vi "Weather API test.vi"() -> ()   [LabVIEW 2019]
uses:
  Source/Open Weather Session/Public/Controls/Weather Data.ctl
  Source/Open Weather Session/Public/Controls/Weather Sample Data.ctl
  Source/Open Weather Session/Public/Controls/Weather Description Data.ctl
  Source/Open Weather Session/Public/Controls/Coordenates.ctl
  Source/Open Weather Session/Open Weather Session.lvclass
panel:
  out "Weather Data":T1
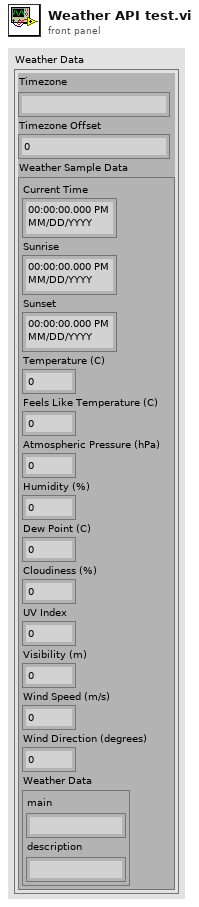
[diagram p1: front panel]
types:
  T1 = typedef "Open Weather Session.lvclass/Weather Data.ctl" = cluster{"Timezone":string, "Timezone Offset":dbl, "Weather Sample Data":T2}
  T2 = typedef "Open Weather Session.lvclass/Weather Sample Data.ctl" = cluster{"Current Time":timestamp, "Sunrise":timestamp, "Sunset":timestamp, "Temperature (C)":dbl, "Feels Like Temperature (C)":dbl, "Atmospheric Pressure (hPa)":dbl, "Humidity (%)":dbl, "Dew Point (C)":dbl, "Cloudiness (%)":dbl, "UV Index":dbl, "Visibility (m)":dbl, "Wind Speed (m/s)":dbl, "Wind Direction (degrees)":dbl, "Weather Data":T3}
  T3 = typedef "Open Weather Session.lvclass/Weather Description Data.ctl" = cluster{"main":string, "description":string}
  T4 = typedef "Open Weather Session.lvclass/Coordenates.ctl" = cluster{"Latitude":dbl, "Longitude":dbl}
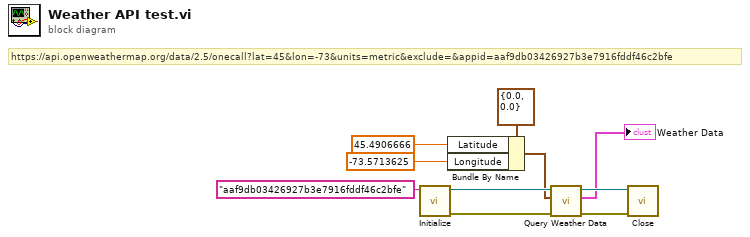
[diagram p0: block diagram]
diagram:
  # "https://api.openweathermap.org/data/2.5/onecall?lat=45&lon=-73&units=metric&exclude=&appid=aaf9db03426927b3e7916fddf46c2bfe"
  n1 = call "Initialize.vi"("API Key"="aaf9db03426927b3e7916fddf46c2bfe" ("input 3")) -> ("Error Out"=w9:errorcluster, "Open Weather Session Out"=w10:refnum<class "Open Weather Session.lvclass">)  [unwired: 9 in]
  n2 = Bundle By Name(cluster=T4 {"Latitude"=0.0, "Longitude"=0.0} ("Coordenates"), "Latitude"=45.4906666 ("input 1"), "Longitude"=-73.5713625 ("input 1")) -> (w3:T4)
  n3 = call-dynamic "Query Weather Data.vi"("Error In"=w9, "Coordenates"=w3, "Open Weather Session In"=w10) -> ("Error Out"=w7:errorcluster, "Weather Data"=→"Weather Data":T1, "Open Weather Session Out"=w8:refnum<class "Open Weather Session.lvclass">)  [unwired: 6 in]
  n4 = call-dynamic "Close.vi"("Error In"=w7, "Open Weather Session In"=w8) -> ()  [unwired: 9 in, 1 out]
